vi "1-5 난수플롯.vi"() -> ()   [LabVIEW 2014]
doc: "이 템플릿을 사용하여 사용자 인터페이스 이벤트 핸들러 디자인 패턴을 생성합니다. 대화 상자 및 다른 사용자 인터페이스에 대하여 이 패턴을 사용합니다. 또한, VI가 사용자 인터페이스 이벤트를 같은 방법으로 다룰 수 있는, 사용자 정의 이벤트를 생성하고 실행할 수 있습니다."
panel:
  in  "탭 컨트롤":enum32{"Setting", "Test"}(tab)
  out "웨이브폼 차트":dbl(graph)
  in  "stop":bool caption="정지"
  in  "Button 1":bool caption="버튼 1"
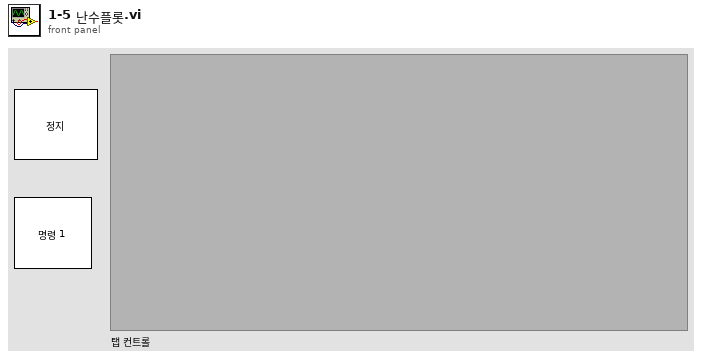
[diagram p1: front panel]
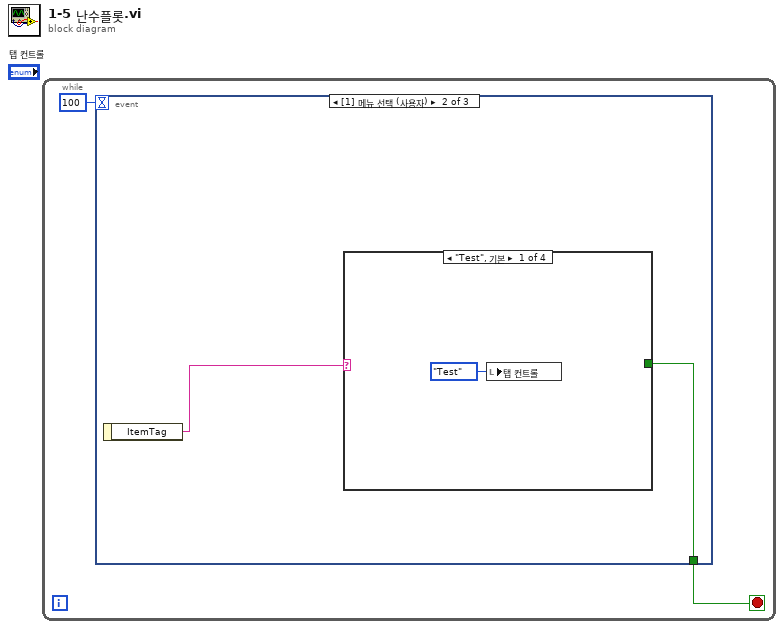
[diagram p0: block diagram]
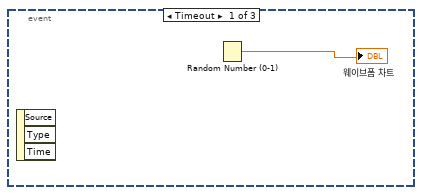
[diagram p2: hidden frame]
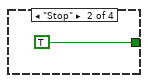
[diagram p3: hidden frame]
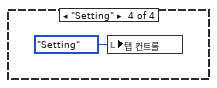
[diagram p5: hidden frame]
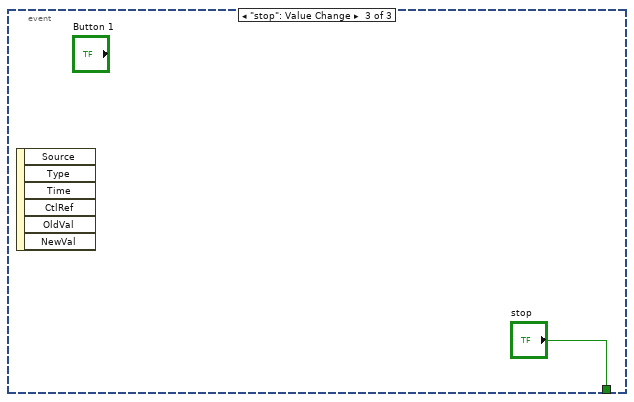
[diagram p6: hidden frame]
diagram:
  n1 = while {
    stop <- w2 stop-if-true
    n2 = event shown="[1] 메뉴 선택 (사용자)" {
      selector: _ -> [_ _ _]
      dyn-events: _ -> [_ _ _]
      timeout: 100 -> [_ _ _]
      tunnel: [_ w4 "stop"] -> w2
      event Timeout {
        n3 = event-data() -> ()  [unwired: 1 in, 3 out]
        n4 = Random Number (0-1)() -> (number: 0 to 1=→"웨이브폼 차트":dbl)
      }
      event Menu Selection (User) {
        n5 = event-data() -> ("ItemTag"=w5:string)  [unwired: 1 in]
        n6 = case shown="\"Test\", 기본" w5 {
          tunnel: [_ TRUE _ _] -> w4
          frame "Test", Default {
            n7 = local write "탭 컨트롤"(enum32{"Setting", "Test"}."Test" ("탭 컨트롤")) -> ()
          }
          frame "Stop" {
          }
          frame "참" {
          }
          frame "Setting" {
            n8 = local write "탭 컨트롤"(enum32{"Setting", "Test"}."Setting" ("탭 컨트롤")) -> ()
          }
        }
      }
      event "stop": Value Change {
        n9 = event-data() -> ()  [unwired: 1 in, 6 out]
      }
    }
  }
